vi "CH_LM Config Trend Time.vi"(0 "Meter Index":i32, 2 "Trend Time (00:01:00)":T1={"Hours"=0, "Minutes"=1, "Seconds"=0}, 3 "Sample Rate /Hz (10Hz)":dbl=10.0 format="%#.3e", 5 "error in (no error)":errorcluster, 7 "Timeout / ms (3000)":i32=3000, 8 "Action (query)":bool, 9 "Lock Timeout / ms (1000)":i32=1000) -> (11 "Lock timed out":bool, 14 "Meter Index":i32, 16 "Trend Time":T1={"Hours"=0, "Minutes"=1, "Seconds"=0}, 17 "Sample Rate / Hz":dbl=10.0 format="%#.3e", 19 "error out":errorcluster)   [LabVIEW 2012, in "CH_LM.lvlib"]
doc: "This command will set/query the trend time and sampling rate, which takes effect at the end of the current trend cycle. The trend cycle duration will be expressed in units of hours:minutes:seconds. \n\nThe sampling interval rate will be expressed in units of samples per seconds. The maximum sampling rate is 10 samples/sec. The true sampling rate will be integer submultiples of 10 samples/sec as the internal probe sampling rate is fixed at exactly 10 samples/sec.\n\n<B>Attention:</B> This command will apply only when a thermopile or optical probe is attached in Watts mode."
uses:
  CH_LM.lvlib
  CH_LM Time.ctl
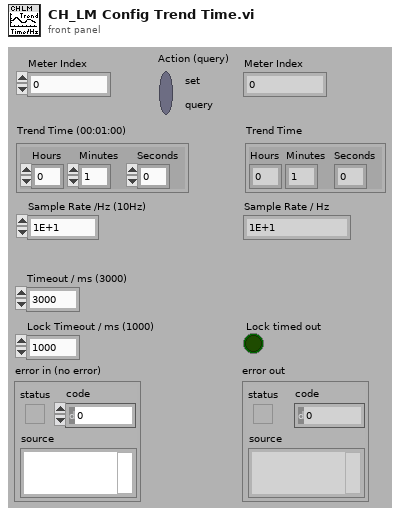
[diagram p1: front panel]
types:
  T1 = typedef "CH_LM.lvlib/CH_LM Time.ctl" = cluster{"Hours":i32, "Minutes":i32, "Seconds":i32}
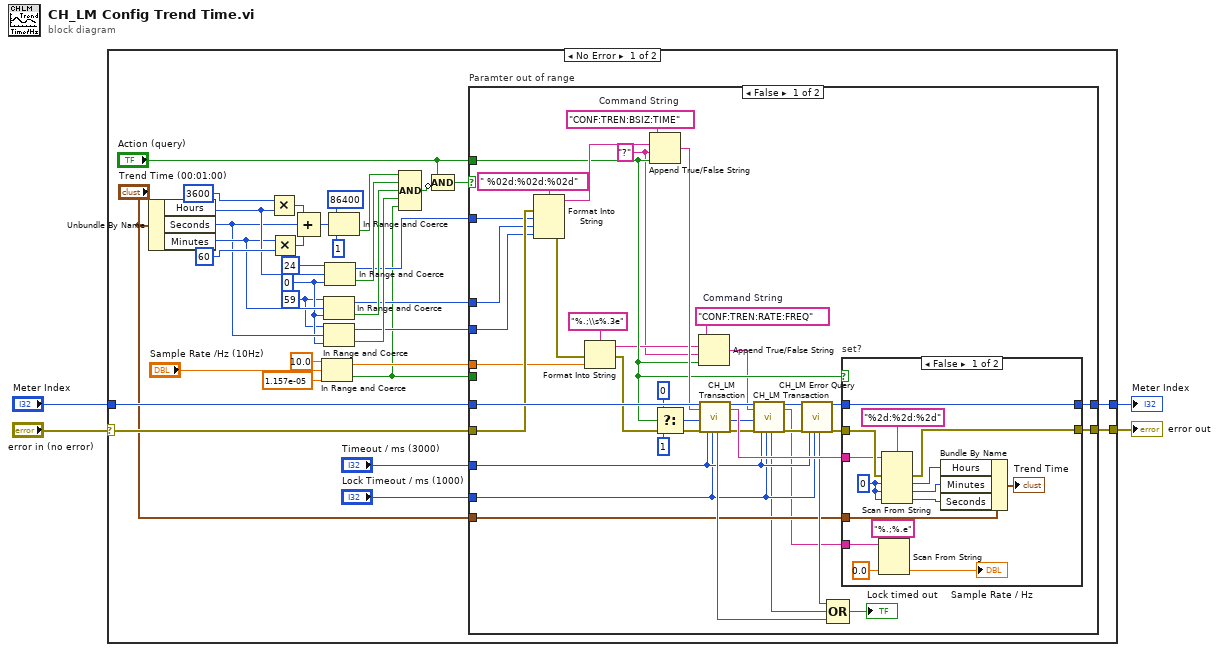
[diagram p0: block diagram]
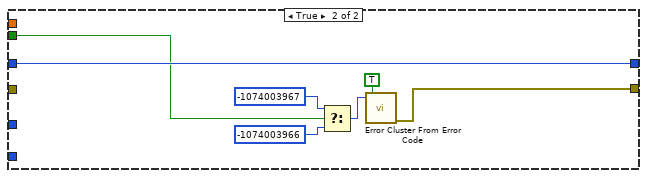
[diagram p3: hidden frame]
diagram:
  n1 = case shown="No Error" "error in (no error)" {
    selector: "error in (no error)" -> [w39 w103]
    tunnel: [w37 w103] -> w4
    tunnel: "Meter Index" -> [w38 w102]
    tunnel: [w36 w102] -> w1
    frame No Error {
      w18 = 59 ("upper limit")
      w19 = 0 ("lower limit")
      n2 = Unbundle By Name("Trend Time (00:01:00)") -> ("Hours"=w22:i32, "Seconds"=w20:i32, "Minutes"=w21:i32)
      n3 = Multiply(x=3600, y=w22) -> (x*y=w28:i32)
      n4 = Multiply(x=w21, y=60) -> (x*y=w27:i32)
      n5 = Compound Arithmetic op=ADD(w28, w20, w27) -> (w26:i32)
      n6 = In Range and Coerce(upper limit=10.0, x="Sample Rate /Hz (10Hz)", lower limit=1.157e-05) -> (coerced(x)=w6:dbl, In Range?=w5:bool)
      n7 = In Range and Coerce(upper limit=w18, x=w21, lower limit=w19) -> (coerced(x)=w11:i32, In Range?=w14:bool)
      n8 = In Range and Coerce(upper limit=w18, x=w20, lower limit=w19) -> (coerced(x)=w10:i32, In Range?=w13:bool)
      n9 = In Range and Coerce(upper limit=24, x=w22, lower limit=w19) -> (coerced(x)=w12:i32, In Range?=w15:bool)
      n10 = In Range and Coerce(upper limit=86400, x=w26, lower limit=1) -> (In Range?=w16:bool)  [unwired: 1 out]
      n11 = Compound Arithmetic op=AND(w16, w15, w14, w13, w5) -> (w17:bool)
      n12 = Compound Arithmetic op=AND("Action (query)", invert w17) -> (w31:bool)
      n13 = case "Paramter out of range" shown="False" w31 {
        tunnel: w39 -> [w65 _]
        tunnel: w38 -> [w77 w101]
        tunnel: [w74 w99] -> w37
        tunnel: [w71 w101] -> w36
        tunnel: "Timeout / ms (3000)" -> [w53 _]
        tunnel: "Lock Timeout / ms (1000)" -> [w52 _]
        tunnel: w12 -> [w62 _]
        tunnel: "Action (query)" -> [w43 _]
        tunnel: "Trend Time (00:01:00)" -> [w58 _]
        tunnel: w11 -> [w60 _]
        tunnel: w10 -> [w59 _]
        tunnel: w6 -> [w46 _]
        tunnel: w5 -> [_ w96]
        frame False {
          w48 = "CONF:TREN:RATE:FREQ"  # Command String
          w41 = "?" ("true string")
          w76 = "CONF:TREN:BSIZ:TIME"  # Command String
          n14 = Format Into String(format string=" %02d:%02d:%02d", error in=w65, w62, w60, w59) -> (resulting string=w63:string, error out=w45:errorcluster)  [unwired: 1 in]
          n15 = Format Into String(format string="%.;\\s%.3e", error in=w45, w46) -> (resulting string=w42:string, error out=w44:errorcluster)  [unwired: 1 in]
          n16 = Append True/False String(1:w43, 2:w41, 3:w63, 4:w76) -> (0:w64:string)
          n17 = Select(t=0, s=w43, f=1 ("NofStrings (-1:all)")) -> (s? t:f=w51:i32)
          n18 = Append True/False String(1:w43, 2:w41, 3:w42, 4:w48) -> (0:w40:string)
          n19 = call "CH_LM Transaction.vi"("Meter Index"=w77, "Command String"=w64, "NofStrings (-1:all)"=w51, "error in (no error)"=w44, "Timeout / ms (3000)"=w53, "Lock Timeout / ms (1000)"=w52) -> ("Lock timed out"=w67:bool, "Meter Index"=w54:i32, "Response"=w75:string, "error out"=w57:errorcluster)  [unwired: 10 out]
          n20 = call "CH_LM Transaction.vi"("Meter Index"=w54, "Command String"=w40, "NofStrings (-1:all)"=w51, "error in (no error)"=w57, "Timeout / ms (3000)"=w53, "Lock Timeout / ms (1000)"=w52) -> ("Lock timed out"=w49:bool, "Meter Index"=w55:i32, "Response"=w50:string, "error out"=w56:errorcluster)  [unwired: 10 out]
          n21 = call "CH_LM Error Query.vi"("Meter Index"=w55, "error in (no error)"=w56, "Timeout / ms (3000)"=w53, "Lock Timeout / ms (1000)"=w52) -> ("Lock timed out"=w68:bool, "Meter Index"=w70:i32, "error out"=w69:errorcluster)  [unwired: 13 out]
          n22 = Compound Arithmetic op=OR(w68, w49, w67) -> (→"Lock timed out":bool)
          n23 = case "set?" shown="False" w43 {
            tunnel: w75 -> [w89 _]
            tunnel: w69 -> [w92 w94]
            tunnel: [w91 w94] -> w74
            tunnel: w70 -> [w90 w93]
            tunnel: [w90 w93] -> w71
            tunnel: w58 -> [w86 _]
            tunnel: w50 -> [w81 _]
            frame False {
              w88 = 0 ("default value 1")
              n24 = Scan From String(format string="%.;%.e", input string=w81, default 1=0.0 ("default value 1")) -> (output 1=→"Sample Rate / Hz":dbl)  [unwired: 2 in, 3 out]
              n25 = Scan From String(format string="%2d:%2d:%2d", input string=w89, error in=w92, default 1=w88, default 2=w88, default 3=w88) -> (error out=w91:errorcluster, output 1=w85:i32, output 2=w84:i32, output 3=w83:i32)  [unwired: 1 in, 2 out]
              n26 = Bundle By Name(cluster=w86, "Hours"=w85, "Minutes"=w84, "Seconds"=w83) -> (→"Trend Time":T1)
            }
            frame True {
            }
          }
        }
        frame True {
          n27 = Select(t=-1074003967 ("error code (0)"), s=w96, f=-1074003966 ("error code (0)")) -> (s? t:f=w97:i32)
          n28 = call <vilib>:"Error Cluster From Error Code.vi"("show call chain? (False)"=TRUE, "error code (0)"=w97) -> ("error out"=w99:errorcluster)  [unwired: 1 in, 6 out]
        }
      }
    }
    frame Error {
    }
  }
  "error out" <- w4
  "Meter Index" <- w1
